vi "Set Acquisiton Time.vi"(4 "error in":errorcluster, 5 "input main cluster":T1, 7 "Acquisition time":dbl) -> (0 "error out":errorcluster, 1 "output main cluster":T1)   [LabVIEW 2010]
uses:
  Main_cluster.ctl
  <vilib>/vision/Image Controls.llb/IMAQ Image.ctl
  C:/Program Files (x86)/National Instruments/LabVIEW 2010/resource/objmgr/daqmx.rc
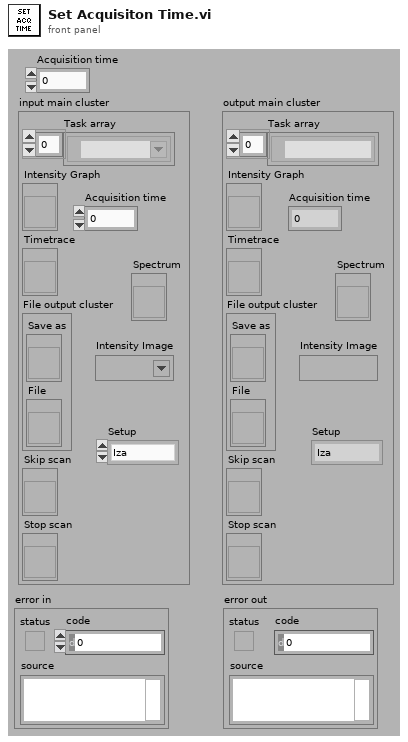
[diagram p1: front panel]
types:
  T1 = typedef "Main_cluster.ctl" = cluster{"Task array":refnum<k21>[], "Intensity Graph":refnum<vi>, "Timetrace":refnum<vi>, "File output cluster":cluster{"Save as":refnum<vi>, "File":refnum<vi>}, "Skip scan":refnum<vi>, "Stop scan":refnum<vi>, "Acquisition time":dbl, "Setup":enum16{"Iza", "Lukasz"}, "Spectrum":refnum<vi>, "Intensity Image":T2}
  T2 = typedef "IMAQ Image.ctl" = refnum<image>
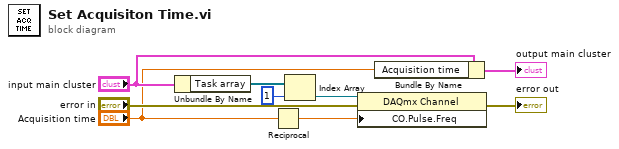
[diagram p0: block diagram]
diagram:
  n1 = Unbundle By Name("input main cluster") -> ("Task array"=w6:refnum<k21>[])
  n2 = Reciprocal(x="Acquisition time") -> (1/x=w7:dbl)
  n3 = Index Array(array=w6, index=1) -> (element=w5:refnum<k21>)
  n4 = property class="DAQmx Channel"(reference=w5, error in="error in", "CO.Pulse.Freq"=w7) -> (error out=→"error out":errorcluster)  [unwired: 1 out]
  n5 = Bundle By Name(cluster="input main cluster", "Acquisition time"="Acquisition time") -> (→"output main cluster":T1)
